vi "Filtering.vi"(10 "order":i32, 11 "Centimeters":dbl) -> (3 "output":dbl)   [LabVIEW 2020]
uses:
  <vilib>/addons/control/pid/pid.llb/PID Control Input Filter (DBL).vi
  <vilib>/addons/control/pid/NI_PID_pid.lvlib
  <vilib>/ptbypt/NI_PtbyPt.lvlib
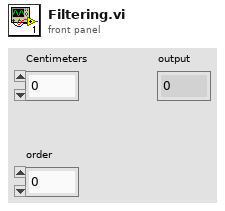
[diagram p1: front panel]
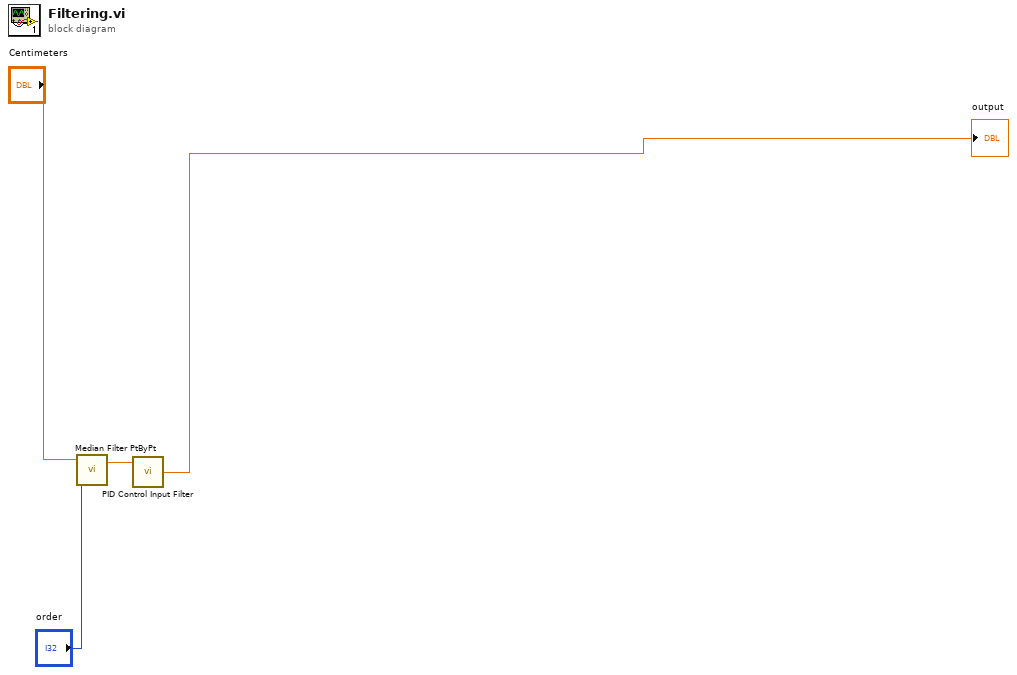
[diagram p0: block diagram]
diagram:
  n1 = call <vilib>:"Median Filter PtByPt.vi"("rank"="order", "x"="Centimeters") -> ("Filtered x"=w1:dbl)  [unwired: 2 in, 1 out]
  n2 = call-poly <vilib>:"PID Control Input Filter.vi"("input"=w1) -> ("output"=→"output":dbl)  [unwired: 4 in]
